vi "FreqCalculation.vi"(3 "Acc Image":T1(plugin-control)) -> (0 "f array":dbl[](array[numeric]))   [LabVIEW 2015]
uses:
  <vilib>/vision/NI_Vision_Development_Module.lvlib
panel:
  out "Histogram Report":T2 {"Standard  Variation" format="%.2f"; "Mean Value" format="%.2f"; "Interval Width" format="%.2f"; "Starting Value" format="%.2f"; "Maximal Value" format="%.2f"; "Minimal Value" format="%.2f"}
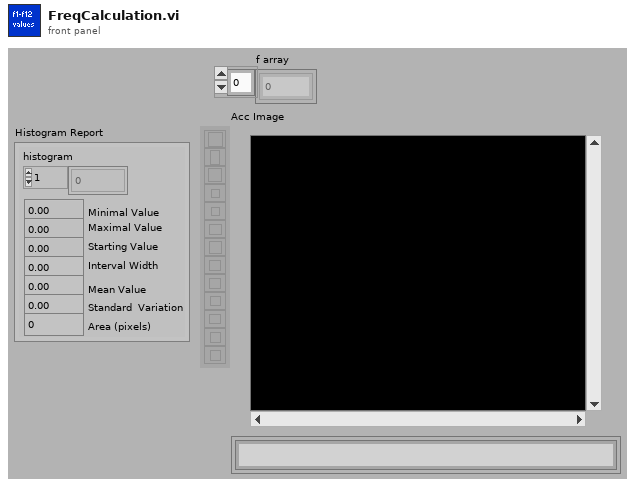
[diagram p1: front panel]
types:
  T1 = typedef "IMAQ Image.ctl" = refnum<image>
  T2 = cluster{"histogram":u32[], "Minimal Value":sgl, "Maximal Value":sgl, "Starting Value":sgl, "Interval Width":sgl, "Mean Value":sgl, "Standard  Variation":sgl, "Area (pixels)":i32}
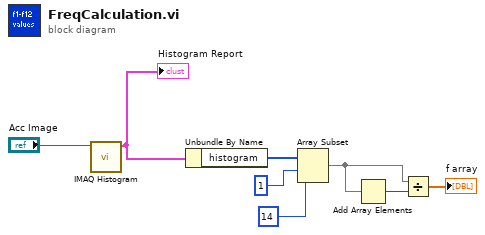
[diagram p0: block diagram]
diagram:
  n1 = call "IMAQ Histogram"("Image"="Acc Image") -> ("Histogram Report"=w8:T2)  [unwired: 4 in, 6 out]
  "Histogram Report" <- w8
  n2 = Unbundle By Name(w8) -> ("histogram"=w7:u32[])
  n3 = Array Subset(array=w7, index=1, length=14) -> (w3:u32[])
  n4 = Add Array Elements(numeric array=w3) -> (sum=w4:u32)
  n5 = Divide(x=w3, y=w4) -> (x/y=→"f array":dbl[])
